vi "Create General Topic.vi"(8 "error in":errorcluster, 9 "Data":variant, 10 "Name":string) -> (0 "error out":errorcluster, 3 "Topic out":refnum<class "Topic.lvclass">)   [LabVIEW 2014, in "Topic.lvclass"]
doc: "This vi is used to create a topic to be passed to the processing loop of the same running client. This is used to \"cut out\" the broker, and all data is kept local to the currently running client."
uses:
  Topic.lvclass
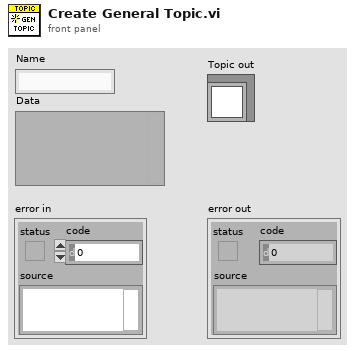
[diagram p1: front panel]
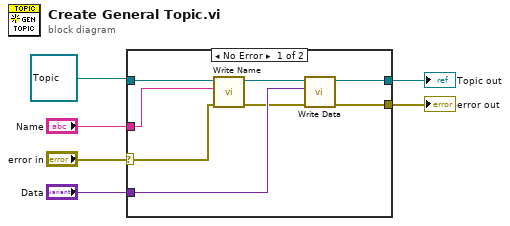
[diagram p0: block diagram]
diagram:
  n1 = case shown="No Error" "error in" {
    selector: "error in" -> [w10 w16]
    tunnel: [w7 w16] -> w5
    tunnel: [w12 w15] -> w4
    tunnel: refnum<class "Topic.lvclass"> refnum ("Topic.lvclass") -> [w14 w15]
    tunnel: "Name" -> [w11 _]
    tunnel: "Data" -> [w9 _]
    frame No Error {
      n2 = call-dynamic "Write Name.vi"("error in"=w10, "Name"=w11, "Topic in"=w14) -> ("error out"=w8:errorcluster, "Topic out"=w13:refnum<class "Topic.lvclass">)  [unwired: 7 in]
      n3 = call-dynamic "Write Data.vi"("error in"=w8, "Data"=w9, "Topic in"=w13) -> ("error out"=w7:errorcluster, "Topic out"=w12:refnum<class "Topic.lvclass">)  [unwired: 7 in]
    }
    frame Error {
    }
  }
  "error out" <- w5
  "Topic out" <- w4
